vi "ROI统计量16bit.vi"(8 "error in (no error)":errorcluster, 9 "ROI Descriptor":T2 {"Contours"."Type" items=["No Selection", "Point", "Line", "Rectangle", "Oval", "Polygon", "Freehand Region", "Annulus", "Unused2", "Unused3", "Broken Line", "Freehand Line", "Rotated Rectangle"]}, 10 "Image Mask":T1, 11 "Image":T1) -> (0 "error out":errorcluster, 2 "统计量":sgl[](array[numeric]), 3 "Image Out":T1)   [LabVIEW 2015]
uses:
  <vilib>/vision/Image Controls.llb/IMAQ Image.ctl
  <vilib>/vision/NI_Vision_Development_Module.lvlib
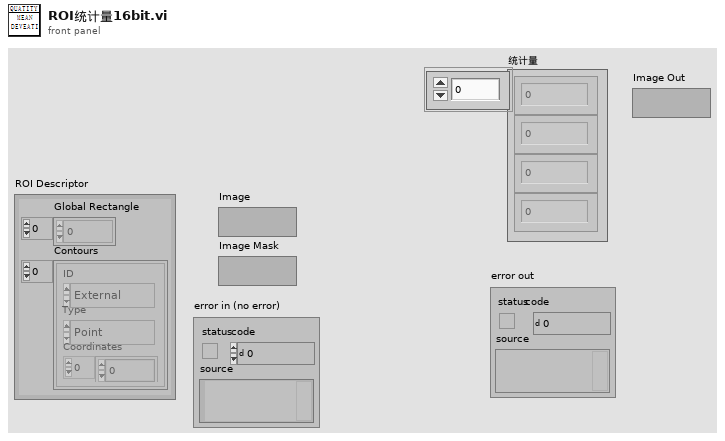
[diagram p1: front panel]
types:
  T1 = typedef "IMAQ Image.ctl" = refnum<image>
  T2 = typedef "ROI Descriptor" = cluster{"Global Rectangle":i32[], "Contours":cluster{"ID":enum32{"External", "Internal"}, "Type":u32, "Coordinates":i32[]}[]}
  T3 = cluster{"Mean Value":sgl, "Standard Variation":sgl, "Minimal Value":sgl, "Maximal Value":sgl, "Area (calibrated)":sgl, "Area (pixels)":i32, "%":sgl}
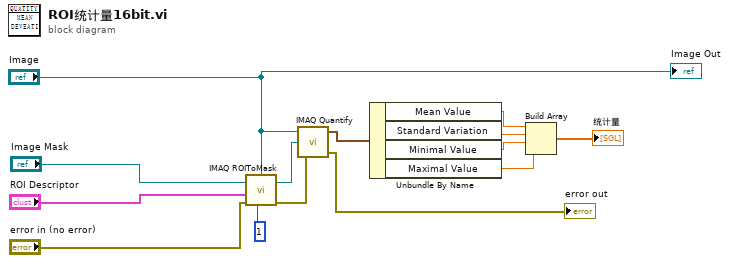
[diagram p0: block diagram]
diagram:
  n1 = call "IMAQ ROIToMask"("error in (no error)"="error in (no error)", "ROI Descriptor"="ROI Descriptor", "Filling Value (255)"=1, "Image"="Image Mask", "Image Model"="Image") -> ("error out"=w8:errorcluster, "Image Out"=w9:T1)  [unwired: 2 out]
  n2 = call "IMAQ Quantify"("error in (no error)"=w8, "Image Mask"=w9, "Image"="Image") -> ("error out"=→"error out":errorcluster, "Global Report"=w14:T3)  [unwired: 1 out]
  n3 = Unbundle By Name(w14) -> ("Mean Value"=w13:sgl, "Standard Variation"=w12:sgl, "Minimal Value"=w11:sgl, "Maximal Value"=w10:sgl)
  n4 = Build Array(w13, w12, w11, w10) -> (→"统计量":sgl[])
  "Image Out" <- "Image"
